vi "Esercitazione 5 - Esercizio per casa, Max e secondo Max Array.vi"() -> ()   [LabVIEW 2018]
panel:
  out "Secondo Massimo":dbl
  out "Massimo":dbl
  in  "Array":dbl[](array[numeric])
  # "dato un array, restituire il massimo E il secondo valore massimo"
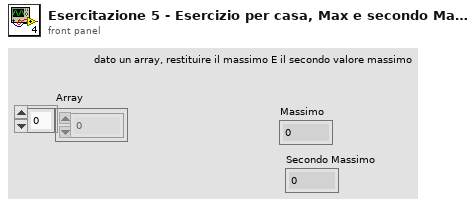
[diagram p1: front panel]
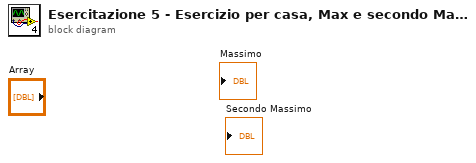
[diagram p0: block diagram]
diagram:
